vi "LNLS Control FOFB Configuration Out.vi"() -> ()   [LabVIEW 2011, in "Controller Global Variables.lvlib"]
uses:
  Controller Global Variables.lvlib
  Types Definitions/Type Control FOFB Configuration Out.ctl
  Types Definitions/Type Operation Mode State.ctl
  Type Definitions.lvlib
panel:
  in  "LNLS Control FOFB Configuration Out":T1={"Status"=0, "Operation Mode"=enum."Manual Mode", "Horizontal Gain"=0.0, "Vertical Gain"=0.0, "Selected Reference Orbit"=0, "Selected Correction Matrix"=0, "Selected FPGA Filters"=0, "Horizontal Distortion Threshold"=0.0, "Vertical Distortion Threshold"=0.0, "Timestamp"=0.0}
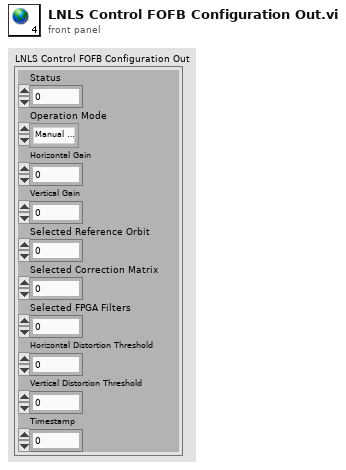
[diagram p1: front panel]
types:
  T1 = typedef "Type Definitions.lvlib/Type Control FOFB Configuration Out.ctl" = cluster{"Status":u16, "Operation Mode":T2, "Horizontal Gain":sgl, "Vertical Gain":sgl, "Selected Reference Orbit":i32, "Selected Correction Matrix":i32, "Selected FPGA Filters":i32, "Horizontal Distortion Threshold":sgl, "Vertical Distortion Threshold":sgl, "Timestamp":dbl}
  T2 = typedef "Type Definitions.lvlib/Type Operation Mode State.ctl" = enum8{"Idle Mode", "Manual Mode", "FOFB Mode"}
diagram:
